vi "Broadcast Refnum Release.vi"(8 "error in":errorcluster) -> (0 "error out":errorcluster)   [LabVIEW 2020, in "SECS Bridge.lvlib"]
uses:
  SECS Bridge.lvlib
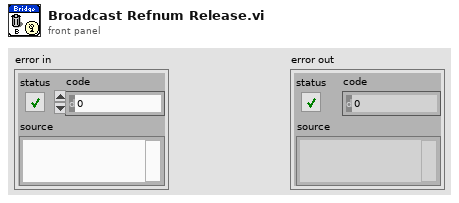
[diagram p1: front panel]
types:
  T1 = typedef "SECS Bridge.lvlib/Broadcast Refnum.ctl" = cluster{"Nottifier Data User Event":refnum<user-event>, "HSMS State User Event":refnum<user-event>, "On-Line User Event":refnum<user-event>}
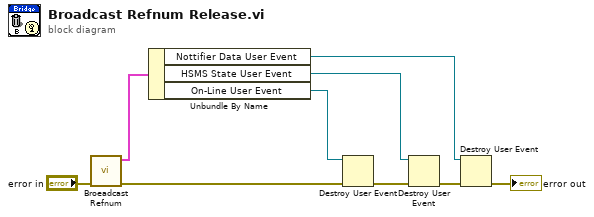
[diagram p0: block diagram]
diagram:
  n1 = call "Broeadcast Refnum.vi"("error in"="error in") -> ("error out"=w3:errorcluster, "Broadcast Refnum"=w6:T1)  [unwired: 9 in]
  n2 = Unbundle By Name(w6) -> ("Nottifier Data User Event"=w8:refnum<user-event>, "HSMS State User Event"=w5:refnum<user-event>, "On-Line User Event"=w2:refnum<user-event>)
  n3 = Destroy User Event(user event=w2, error in=w3) -> (error out=w1:errorcluster)
  n4 = Destroy User Event(user event=w5, error in=w1) -> (error out=w4:errorcluster)
  n5 = Destroy User Event(user event=w8, error in=w4) -> (error out=→"error out":errorcluster)
